vi "Convert I2C Messages & Buffer U8.vi"(8 "error in (no error)":errorcluster, 10 "STREAMING Ref":refnum<vi>, 11 "Data":u8[](array[numeric])) -> (0 "error out":errorcluster)   [LabVIEW 2025, in "I2C Bus Monitor UI.lvlib"]
uses:
  I2C Bus Monitor UI.lvlib
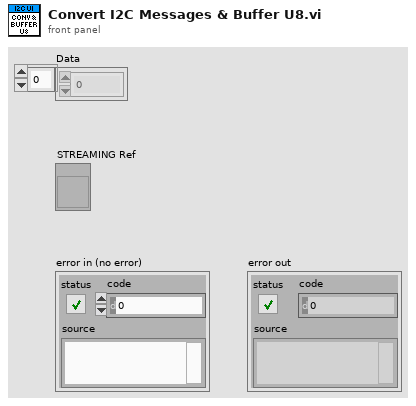
[diagram p1: front panel]
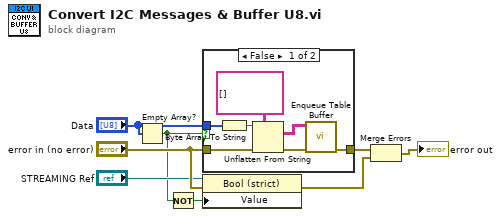
[diagram p0: block diagram]
diagram:
  n1 = Empty Array?(array="Data") -> (empty?=w5:bool)
  n2 = Not(x=w5) -> (.not. x?=w4:bool)
  n3 = case shown="False" w5 {
    tunnel: "error in (no error)" -> [w10 w16]
    tunnel: "Data" -> [w13 _]
    tunnel: [w11 w16] -> w7
    frame False {
      n4 = Byte Array To String(unsigned byte array=w13) -> (string=w14:string)
      n5 = Unflatten From String(type=string[][] [] ("Fetched I2C Messages"), binary string=w14, error in (no error)=w10) -> (value=w9:string[][], error out=w12:errorcluster)  [unwired: 2 in, 1 out]
      n6 = call "Enqueue Table Buffer.vi"("error in (no error)"=w12, "Data"=w9) -> ("error out"=w11:errorcluster)  [unwired: 9 in]
    }
    frame True {
    }
  }
  n7 = property class="Bool (strict)"(reference="STREAMING Ref", error in="error in (no error)", "Value"=w4) -> (error out=w2:errorcluster)  [unwired: 1 out]
  n8 = Merge Errors(w7, w2) -> (→"error out":errorcluster)
